vi "THFLSHdll_d.vi"(5 "dll_path_in":path, 6 "i":dbl, 8 "error in (no error)":errorcluster, 9 "Component Molar Fractions":dbl[](array[numeric])=[1.0, 0.0, 0.0, 0.0, 0.0, 0.0, 0.0, 0.0, 0.0, 0.0, 0.0, 0.0, 0.0, 0.0, 0.0, 0.0, 0.0, 0.0, 0.0, 0.0], 10 "h":dbl, 11 "Temp (deg c)":dbl=30.0) -> (0 "error out":errorcluster, 3 "THDATAOUT":dbl[](array[numeric]), 4 "dll_path_out":path)   [LabVIEW 2017]
doc: "Please feel free to contact me if you have any questions .\nMy mail:ken_pop@tom.com yan.ding@jci.com"
panel:
  out "x":dbl[](array[numeric])
  out "d":dbl
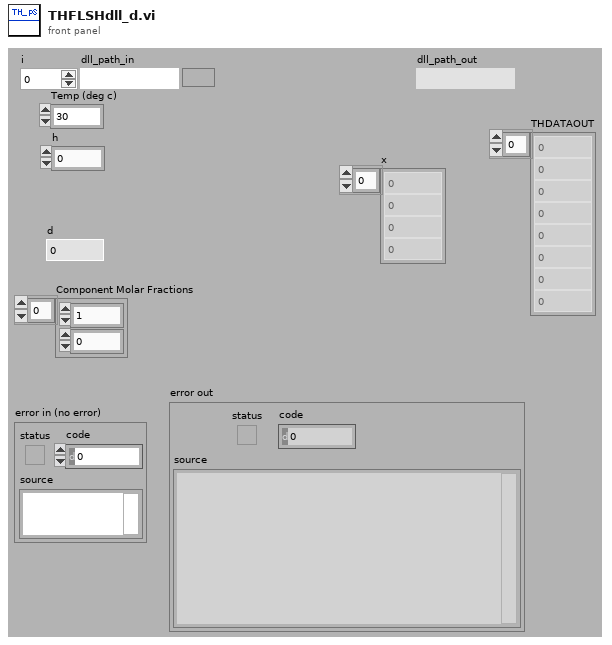
[diagram p1: front panel]
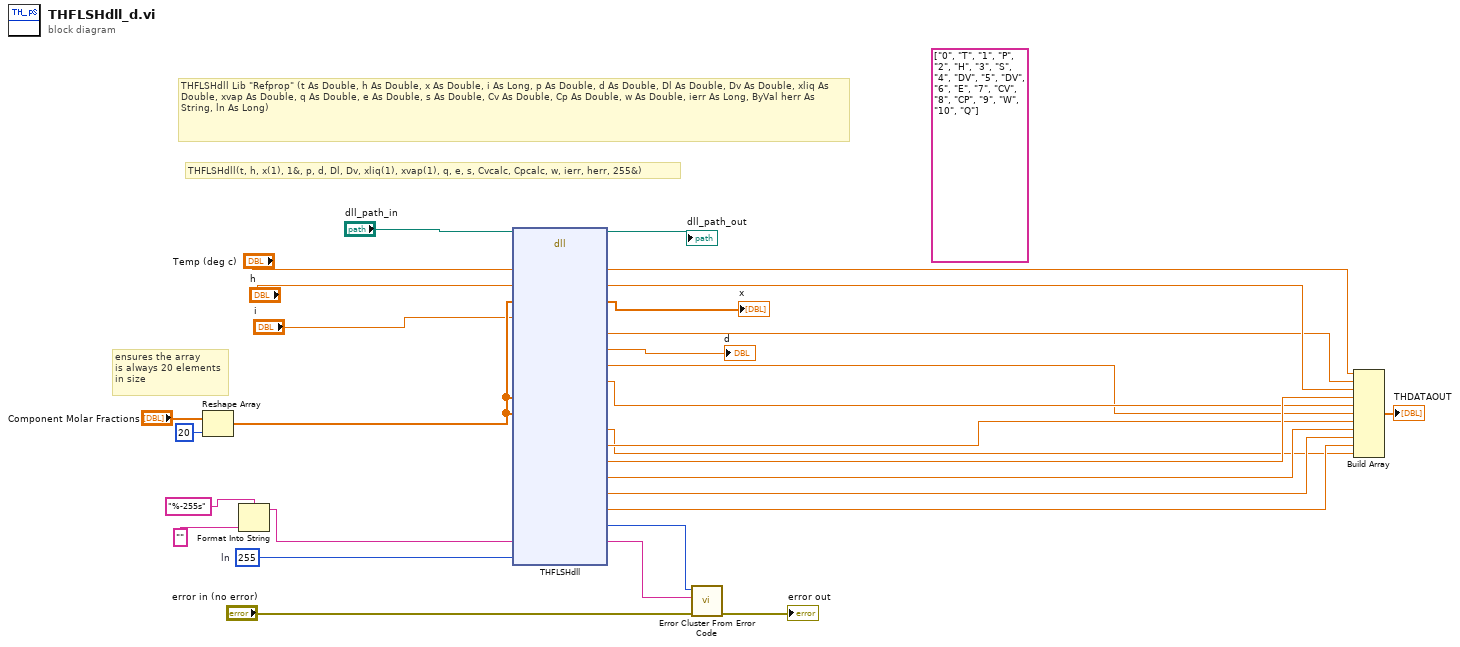
[diagram p0: block diagram]
diagram:
  (unwired) string[][] [["0", "T"], ["1", "P"], ["2", "H"], ["3", "S"], ["4", "DV"], ["5", "DV"], ["6", "E"], ["7", "CV"], ["8", "CP"], ["9", "W"], ["10", "Q"]] ("数组")
  w22 = 255  # ln
  # "THFLSHdll(t, h, x(1), 1&, p, d, Dl, Dv, xliq(1), xvap(1), q, e, s, Cvcalc, Cpcalc, w, ierr, herr, 255&)"
  # "THFLSHdll Lib \"Refprop\" (t As Double, h As Double, x As Double, i As Long, p As Double, d As Double, Dl As Double, Dv As Double, xliq As Double, xvap As Double, q As Double, e As Double, s As Double, Cv As Double, Cp As Double, w As Double, ierr As Long, ByVal herr As String, ln As Long)"
  # "ensures the array\nis always 20 elements\nin size"
  n1 = Reshape Array("Component Molar Fractions", 20 ("dimension size")) -> (w18:dbl[])
  n2 = Format Into String(format string="%-255s", "") -> (resulting string=w21:string)  [unwired: 2 in, 1 out]
  n3 = dll-call lib="refprop.DLL" fn="THFLSHdll"(path in="dll_path_in", "t"="Temp (deg c)", "h"="h", "x"=w18, "i"="i", "xliq"=w18, "xvap"=w18, "herr"=w21, "ln"=w22) -> (path out=→"dll_path_out":path, "t"=w14:dbl, "h"=w13:dbl, "x"=→"x":dbl[], "p"=w4:dbl, "d"=→"d":dbl, "Dl"=w10:dbl, "Dv"=w11:dbl, "q"=w5:dbl, "e"=w9:dbl, "s"=w12:dbl, "cv"=w8:dbl, "cp"=w7:dbl, "w"=w6:dbl, "ierr"=w23:i32, "herr"=w24:string)  [unwired: 18 in, 1 out]
  n4 = call <vilib>:"Error Cluster From Error Code.vi"("error in (no error)"="error in (no error)", "error message (\"\")"=w24, "error code (0)"=w23) -> ("error out"=→"error out":errorcluster)  [unwired: 6 in]
  n5 = Build Array(w14, w4, w13, w12, w11, w10, w9, w8, w7, w6, w5) -> (→"THDATAOUT":dbl[])
